vi "Test2.vi"() -> ()   [LabVIEW 2020]
uses:
  Postgres Connector/Cluster_Return_Of_The_Query.ctl
  Postgres Connector/Postgres Connector.lvclass
panel:
  out "Query Return":T1[](array[typedef])
  in  "Connection Info":T2={"IP Address"="192.168.5.50", "Port"=5432, "Timeout"=2000, "User"="postgres", "Password"="28779867", "Database"="postgres"}
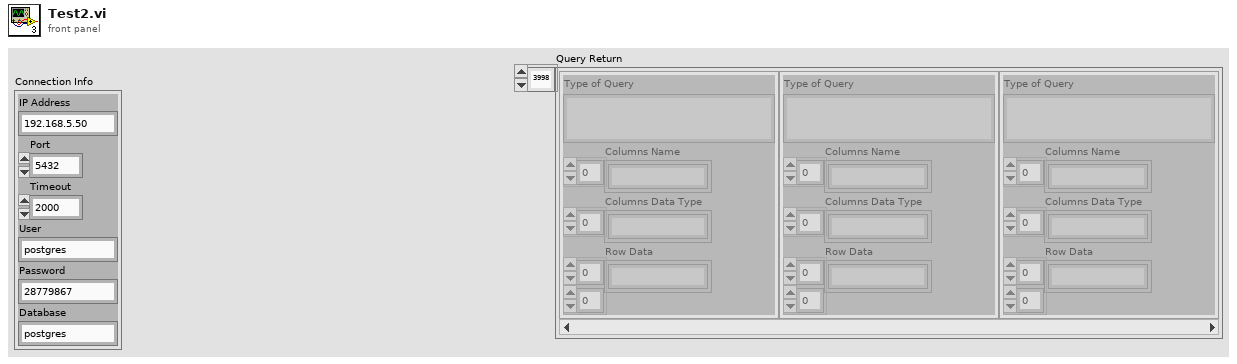
[diagram p1: front panel]
types:
  T1 = typedef "Postgres Connector.lvclass/Cluster_Return_Of_The_Query.ctl" = cluster{"Type of Query":string, "Columns Name":string[], "Columns Data Type":string[], "Row Data":string[][]}
  T2 = cluster{"IP Address":string, "Port":u16, "Timeout":i32, "User":string, "Password":string, "Database":string}
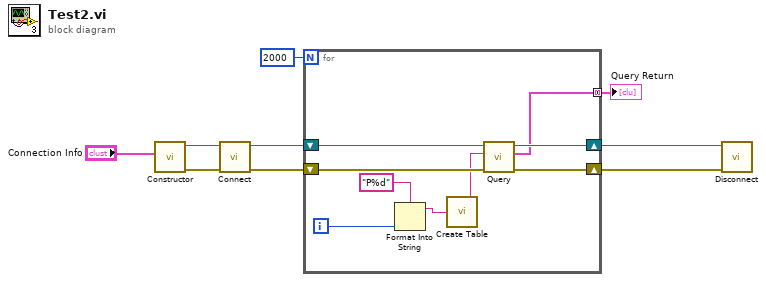
[diagram p0: block diagram]
diagram:
  n1 = call "Constructor.vi"("Connection Info"="Connection Info") -> ("error out"=w8:errorcluster, "Postgres Connector Out"=w7:refnum<class "Postgres Connector.lvclass">)  [unwired: 9 in]
  n2 = call "Connect.vi"("error in (no error)"=w8, "Postgres Connector In"=w7) -> ("error out"=w6:errorcluster, "Postgres Connector Out"=w5:refnum<class "Postgres Connector.lvclass">)  [unwired: 8 in]
  n3 = for {
    N: 2000 -> [_]
    shift-right: [w15] -> w3
    shift-left: w6 -> [w18]
    shift-right: [w16] -> w4
    shift-left: w5 -> [w17]
    tunnel: [w10] -> w1 mode=concatenating
    i -> [w14]
    n4 = Format Into String(format string="P%d", w14) -> (resulting string=w12:string)  [unwired: 2 in, 1 out]
    n5 = call "Create Table.vi"("Table Name"=w12) -> ("resulting string"=w11:string)
    n6 = call "Query.vi"("error in (no error)"=w18, "Query"=w11, "Postgres Connector In"=w17) -> ("error out"=w15:errorcluster, "Query Return"=w10:T1[], "Postgres Connector Out"=w16:refnum<class "Postgres Connector.lvclass">)  [unwired: 6 in]
  }
  "Query Return" <- w1
  n7 = call "Disconnect.vi"("error in (no error)"=w3, "Postgres Connector In"=w4) -> ()  [unwired: 8 in, 2 out]
